vi "Read Analogue.vi"(8 "error in (no error)":errorcluster, 11 "Sim HiPOT in":refnum<class "Sim HiPOT.lvclass">) -> (0 "error out":errorcluster, 2 "Measurements":dbl, 3 "Sim HiPOT out":refnum<class "Sim HiPOT.lvclass">)   [LabVIEW 2021, in "Concrete.lvlib" / "Sim HiPOT.lvclass"]
uses:
  Sim HiPOT.lvclass
  <vilib>/numeric/Random Number (Range) DBL.vi
  Harware Abstraction/HiPOT/HiPOT.lvclass
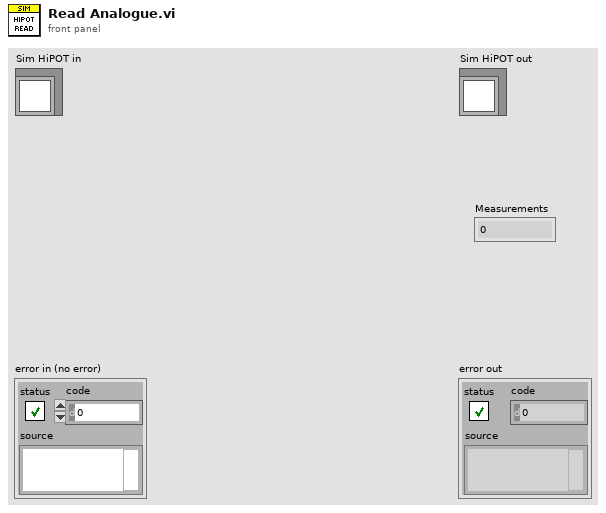
[diagram p1: front panel]
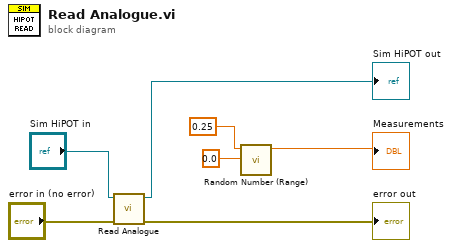
[diagram p0: block diagram]
diagram:
  n1 = call-parent "Read Analogue.vi"("error in (no error)"="error in (no error)", "PS in"="Sim HiPOT in") -> ("error out"=→"error out":errorcluster, "PS out"=→"Sim HiPOT out":refnum<class "Sim HiPOT.lvclass">)  [unwired: 7 in, 1 out]
  n2 = call-poly <vilib>:"Random Number (Range).vi"("lower bound (0)"=0.0, "upper bound (100)"=0.25) -> ("number"=→"Measurements":dbl)  [unwired: 9 in]
